vi "PUT X Position Data.vi"(0 "X Position Data":dbl[](array[numeric])) -> ()   [LabVIEW 2013]
uses:
  Functional Globals/Action.ctl
  Interpreted Data FGV Selector.ctl
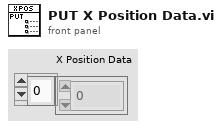
[diagram p1: front panel]
types:
  T1 = typedef "Interpreted Data FGV Selector.ctl" = enum16{"X Position", "Y Position", "Z Position", "Force", "Signal Strength"}
  T2 = typedef "Action.ctl" = enum16{"GET", "PUT", "DELETE"}
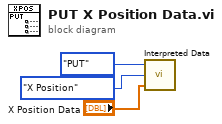
[diagram p0: block diagram]
diagram:
  n1 = call "Interpreted Data.vi"("Input"="X Position Data", "Interpreted Data FGV Selector"=Interpreted_Data_FGV_Selector."X Position", "Action"=Action."PUT") -> ()  [unwired: 2 in, 1 out]
